vi "AssertDisable.vi"(0 "VI Reference In":refnum<vi>, 1 "Label (VI Title)":string="Default", 11 "error in (no error)":errorcluster) -> (4 "VI Reference Out":refnum<vi>, 15 "error out":errorcluster)   [LabVIEW 2016, in "DronaTest.lvlib"]
uses:
  DronaTest.lvlib
  main/apis/Stimulus/ValueSignal/ValueSignalByPathString.vi
  main/apis/Assert/AssertControlDisable/AssertDisabled.vi
  main/apis/Assert/AssertControlDisable/AssertDisabledAndGrayedOut.vi
  main/apis/Assert/AssertControlDisable/AssertEnabled.vi
  <vilib>/addons/_JKI Toolkits/Caraya/classes/Assert/Assert Not Error.vi
  <vilib>/addons/_JKI Toolkits/Caraya/classes/Test/Test.lvclass
  main/Drona.lvlib
  <vilib>/addons/_JKI Toolkits/Caraya/classes/Assert/Assert.lvclass
  main/apis/Assert/AssertControlDisable/AssertControlDisable.lvlib
  main/apis/Stimulus/ValueSignal/ValueSignal.lvlib
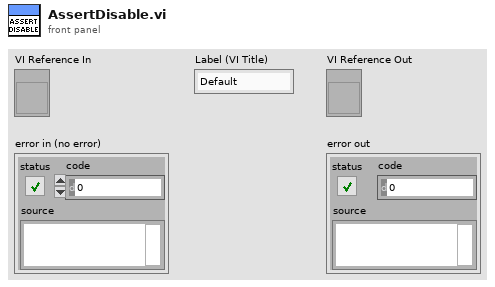
[diagram p1: front panel]
types:
  T1 = enum8{"Enabled", "Disabled", "Disabled and Grayed Out"}
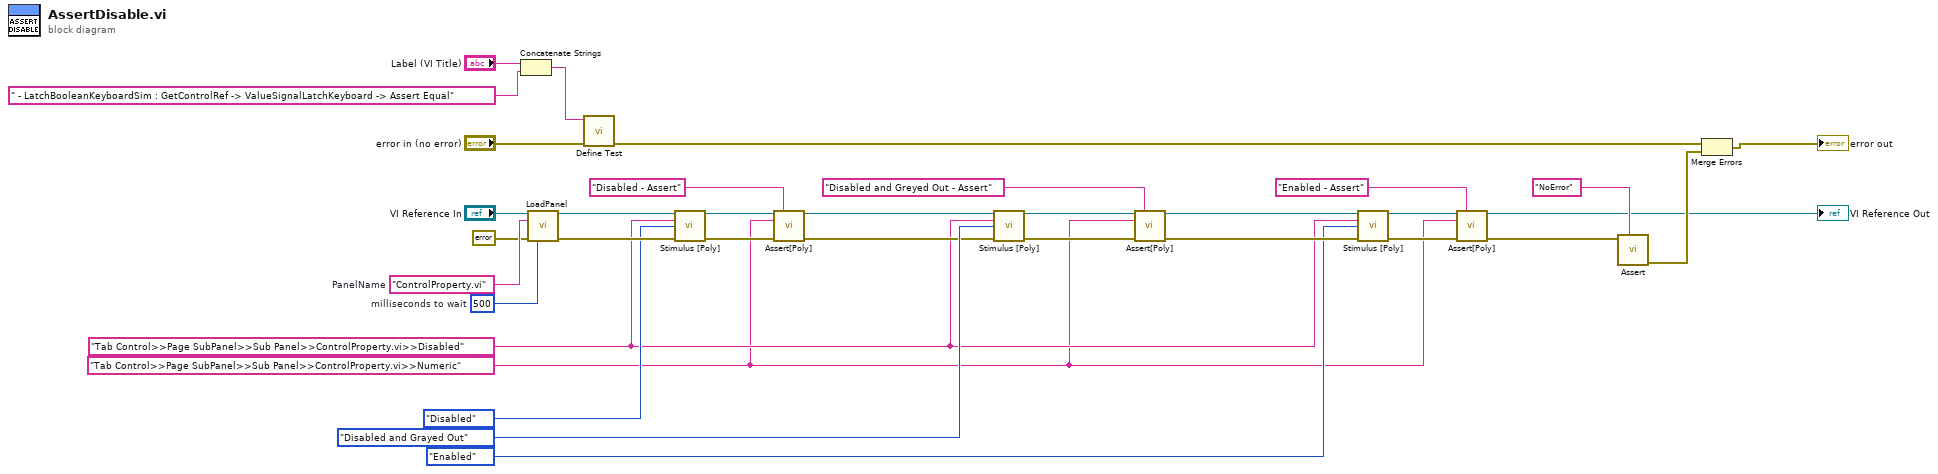
[diagram p0: block diagram]
diagram:
  w18 = u32 500  # milliseconds to wait
  w1 = "Tab Control>>Page SubPanel>>Sub Panel>>ControlProperty.vi>>Numeric" ("Control Path")
  w2 = "Tab Control>>Page SubPanel>>Sub Panel>>ControlProperty.vi>>Disabled" ("Control Path")
  w26 = "ControlProperty.vi"  # PanelName
  n1 = Concatenate Strings("Label (VI Title)", " - LatchBooleanKeyboardSim : GetControlRef -> ValueSignalLatchKeyboard -> Assert Equal" ("Label (VI Title)")) -> (w28:string)
  n2 = call "LoadPanel.vi"("VI in"="VI Reference In", "Panel Name"=w26, "error in (no error)"=errorcluster {"status"=FALSE, "code"=0, "source"=""} ("error in"), "milliseconds to wait"=w18) -> ("VI out"=w23:refnum<vi>, "error out"=w20:errorcluster)  [unwired: 10 in]
  n3 = call <vilib>:"Define Test.vi"("error in (no error)"="error in (no error)", "Label (VI Title)"=w28) -> ("error out"=w31:errorcluster)  [unwired: 9 in]
  n4 = call-poly "Stimulus [Poly].vi"("VI Reference In"=w23, "Control Path"=w2, "Value (Signaling)"=T1."Disabled" ("Disabled"), "error in"=w20) -> ("VI Reference Out"=w22:refnum<vi>, "error out"=w24:errorcluster)  [unwired: 10 in]
  n5 = call-poly "Assert[Poly].vi"("VI Reference In"=w22, "Label"="Disabled - Assert" ("string"), "Control Path"=w1, "Error In"=w24) -> ("VI Reference Out"=w12:refnum<vi>, "Error Out"=w11:errorcluster)  [unwired: 10 in]
  n6 = call-poly "Stimulus [Poly].vi"("VI Reference In"=w12, "Control Path"=w2, "Value (Signaling)"=T1."Disabled and Grayed Out" ("Disabled"), "error in"=w11) -> ("VI Reference Out"=w14:refnum<vi>, "error out"=w13:errorcluster)  [unwired: 10 in]
  n7 = call-poly "Assert[Poly].vi"("VI Reference In"=w14, "Label"="Disabled and Greyed Out - Assert" ("string"), "Control Path"=w1, "Error In"=w13) -> ("VI Reference Out"=w6:refnum<vi>, "Error Out"=w7:errorcluster)  [unwired: 10 in]
  n8 = call-poly "Stimulus [Poly].vi"("VI Reference In"=w6, "Control Path"=w2, "Value (Signaling)"=T1."Enabled" ("Disabled"), "error in"=w7) -> ("VI Reference Out"=w9:refnum<vi>, "error out"=w10:errorcluster)  [unwired: 10 in]
  n9 = call-poly "Assert[Poly].vi"("VI Reference In"=w9, "Label"="Enabled - Assert" ("string"), "Control Path"=w1, "Error In"=w10) -> ("VI Reference Out"=→"VI Reference Out":refnum<vi>, "Error Out"=w4:errorcluster)  [unwired: 10 in]
  n10 = call-poly <vilib>:"Assert.vi"("Label"="NoError" ("string"), "Not Error?"=w4) -> ("error out"=w34:errorcluster)  [unwired: 9 in]
  n11 = Merge Errors(w31, w34) -> (→"error out":errorcluster)
